vi "ClusterFourChannels.vi"(5 "Trace3":u8, 6 "binning (s)":dbl format="%.8f", 7 "Trace 2":u8=2, 8 "Trace 1":u8=3, 9 "Trace 0":u8=4, 10 "MCS":u32[][](array[numeric])) -> (0 "channel 3":cluster{i32, "binning (s)":dbl, "MCS":u32[]} {"binning (s)" format="%.2f"}, 1 "channel 2":T1 {"binning (s)" format="%.2f"; "offset" format="%.2f"}, 2 "channel 1":T1 {"binning (s)" format="%.2f"; "offset" format="%.2f"}, 3 "channel 0":T1 {"binning (s)" format="%.2f"; "offset" format="%.2f"}, 4 "sum":T1 {"binning (s)" format="%.2f"; "offset" format="%.2f"})   [LabVIEW 2009]
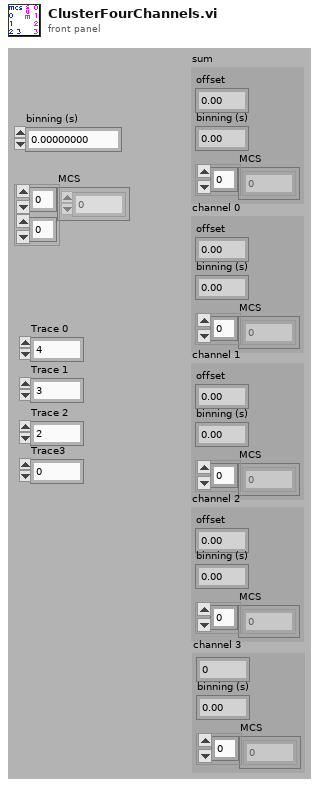
[diagram p1: front panel]
types:
  T1 = cluster{"offset":dbl, "binning (s)":dbl, "MCS":u32[]}
  T2 = cluster{" offset ":i32, "binning (s)":dbl, "MCS":u32[]}
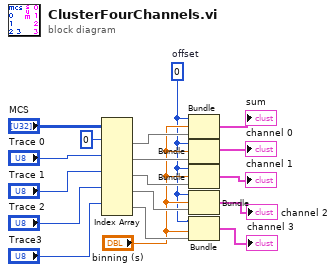
[diagram p0: block diagram]
diagram:
  w2 = 0  # offset
  n1 = Index Array(array="MCS", index (row) #1=0 ("index (row)"), index (row) #2="Trace 0", index (row) #3="Trace 1", index (row) #4="Trace 2", index (row) #5="Trace3") -> (element #1=w17:u32[], element #2=w15:u32[], element #3=w13:u32[], element #4=w8:u32[], element #5=w4:u32[])  [unwired: 5 in]
  n2 = Bundle("offset"=w2, "binning (s)"="binning (s)", "MCS"=w17) -> (→"sum":T2)  [unwired: 1 in]
  n3 = Bundle("offset"=w2, "binning (s)"="binning (s)", "MCS"=w15) -> (→"channel 0":T2)  [unwired: 1 in]
  n4 = Bundle("offset"=w2, "binning (s)"="binning (s)", "MCS"=w13) -> (→"channel 1":T2)  [unwired: 1 in]
  n5 = Bundle("offset"=w2, "binning (s)"="binning (s)", "MCS"=w8) -> (→"channel 2":T2)  [unwired: 1 in]
  n6 = Bundle("offset"=w2, "binning (s)"="binning (s)", "MCS"=w4) -> (→"channel 3":T2)  [unwired: 1 in]
